vi "InputProc.vi"(7 "error in":errorcluster, 8 "output cluster":T15={[], {[], [], [], "GyroDevRef"={"DevStatus"={"status"=FALSE, "code"=0, "source"=""}, "Analog Channel"=enum."AI 0", "Offset"=0.0, "Gain (VoltsPerDegree/Second)"=0.0, "Gyro Type"=enum."Analog", "Handle"=0, "SPI Bus"=enum."Invalid", "Device Found"=FALSE, "Sample Rate"=1.0, "Calibrate On Open"=FALSE}, "CompressorDevRef"={"DevStatus"={"status"=FALSE, "code"=0, "source"=""}, "Pneumatics Control Module"=0}}} {"?"."GyroDevRef"."Sample Rate" min=0.25 max=100.0 step=0.25}, 9 "SensorInputData":T16, 10 "GamepadData":T17) -> (0 "error out":errorcluster, 2 "SensorInputDataOut":T16, 3 "GamepadDataOut":T17)   [LabVIEW 2015]
uses:
  Typedefs/GamepadData.ctl
  Typedefs/SensorInputData.ctl
  <vilib>/Rock Robotics/WPI/Joystick/WPI_JoystickDevRef.ctl
  <vilib>/Rock Robotics/WPI/Joystick/WPI_JoystickDeviceEnum.ctl
  <vilib>/Rock Robotics/WPI/Potentiometer/WPI_PotentiometerDevRef.ctl
  <vilib>/Rock Robotics/SystemInterfaces/AI/FPGA_AIChannel.ctl
  <vilib>/Rock Robotics/WPI/Encoder/WPI_EncoderDevRef.ctl
  <vilib>/Rock Robotics/SystemInterfaces/Encoder/FPGA_EncoderIdx.ctl
  <vilib>/Rock Robotics/SystemInterfaces/Counter/FPGA_CounterCtrSystemIndex.ctl
  <vilib>/Rock Robotics/WPI/Encoder/WPI_EncoderType.ctl
  <vilib>/Rock Robotics/WPI/Switch/WPI_SwitchDevRef.ctl
  <vilib>/Rock Robotics/SystemInterfaces/DIO/FPGA_DIOChannel.ctl
  <vilib>/Rock Robotics/WPI/Gyro/WPI_GyroDevRef.ctl
  <vilib>/Rock Robotics/SystemInterfaces/spilib/spi_bus.ctl
  <vilib>/Rock Robotics/WPI/Compressor/WPI_CompressorDevRef.ctl
  Gensubs/Bert_or_Ernie.vi
  Typedefs/JoysticksGlobal.vi
panel:
  in  "Wench Deadzone Limit":dbl=0.05 format="%#_13g"
  in  "X360 Deadzone Limit":dbl=0.3
  in  "Bert Arm Inputs":T1={"SensorMax"=0.929, "UnitMin"=-26.5, "SensorMin"=0.502, "UnitMax"=86.8}
  in  "Ernie Arm Inputs":T1={"SensorMax"=0.837, "UnitMin"=-26.7, "SensorMin"=0.444, "UnitMax"=87.4}
  out "Claw Pot Raw":dbl
  in  "Ernie StackerClamp Inputs":T1={"SensorMax"=0.852, "UnitMin"=148.3, "SensorMin"=0.477, "UnitMax"=219.6}
  in  "Ernie Stacker Inputs":T1={"SensorMax"=0.782, "UnitMin"=0.0, "SensorMin"=0.357, "UnitMax"=21.125}
  in  "Bert StackerClamp Inputs":T1={"SensorMax"=0.42, "UnitMin"=141.5, "SensorMin"=0.064, "UnitMax"=217.6}
  out "Stacker Clamp Pot Raw":dbl format="%#_13g"
  in  "F310 Deadzone Limit":dbl=0.05
  out "Arm Pot Raw":dbl
  out "Stacker Pot Raw":dbl
  in  "Bert Stacker Inputs":T1={"SensorMax"=0.501, "UnitMin"=0.0, "SensorMin"=0.082, "UnitMax"=21.125}
  in  "ENC_CPI":dbl=0.145
  # "is now f310"
  # "ENC_CPI is encoder counts per inch"
  # "Analog"
  # "XRS"
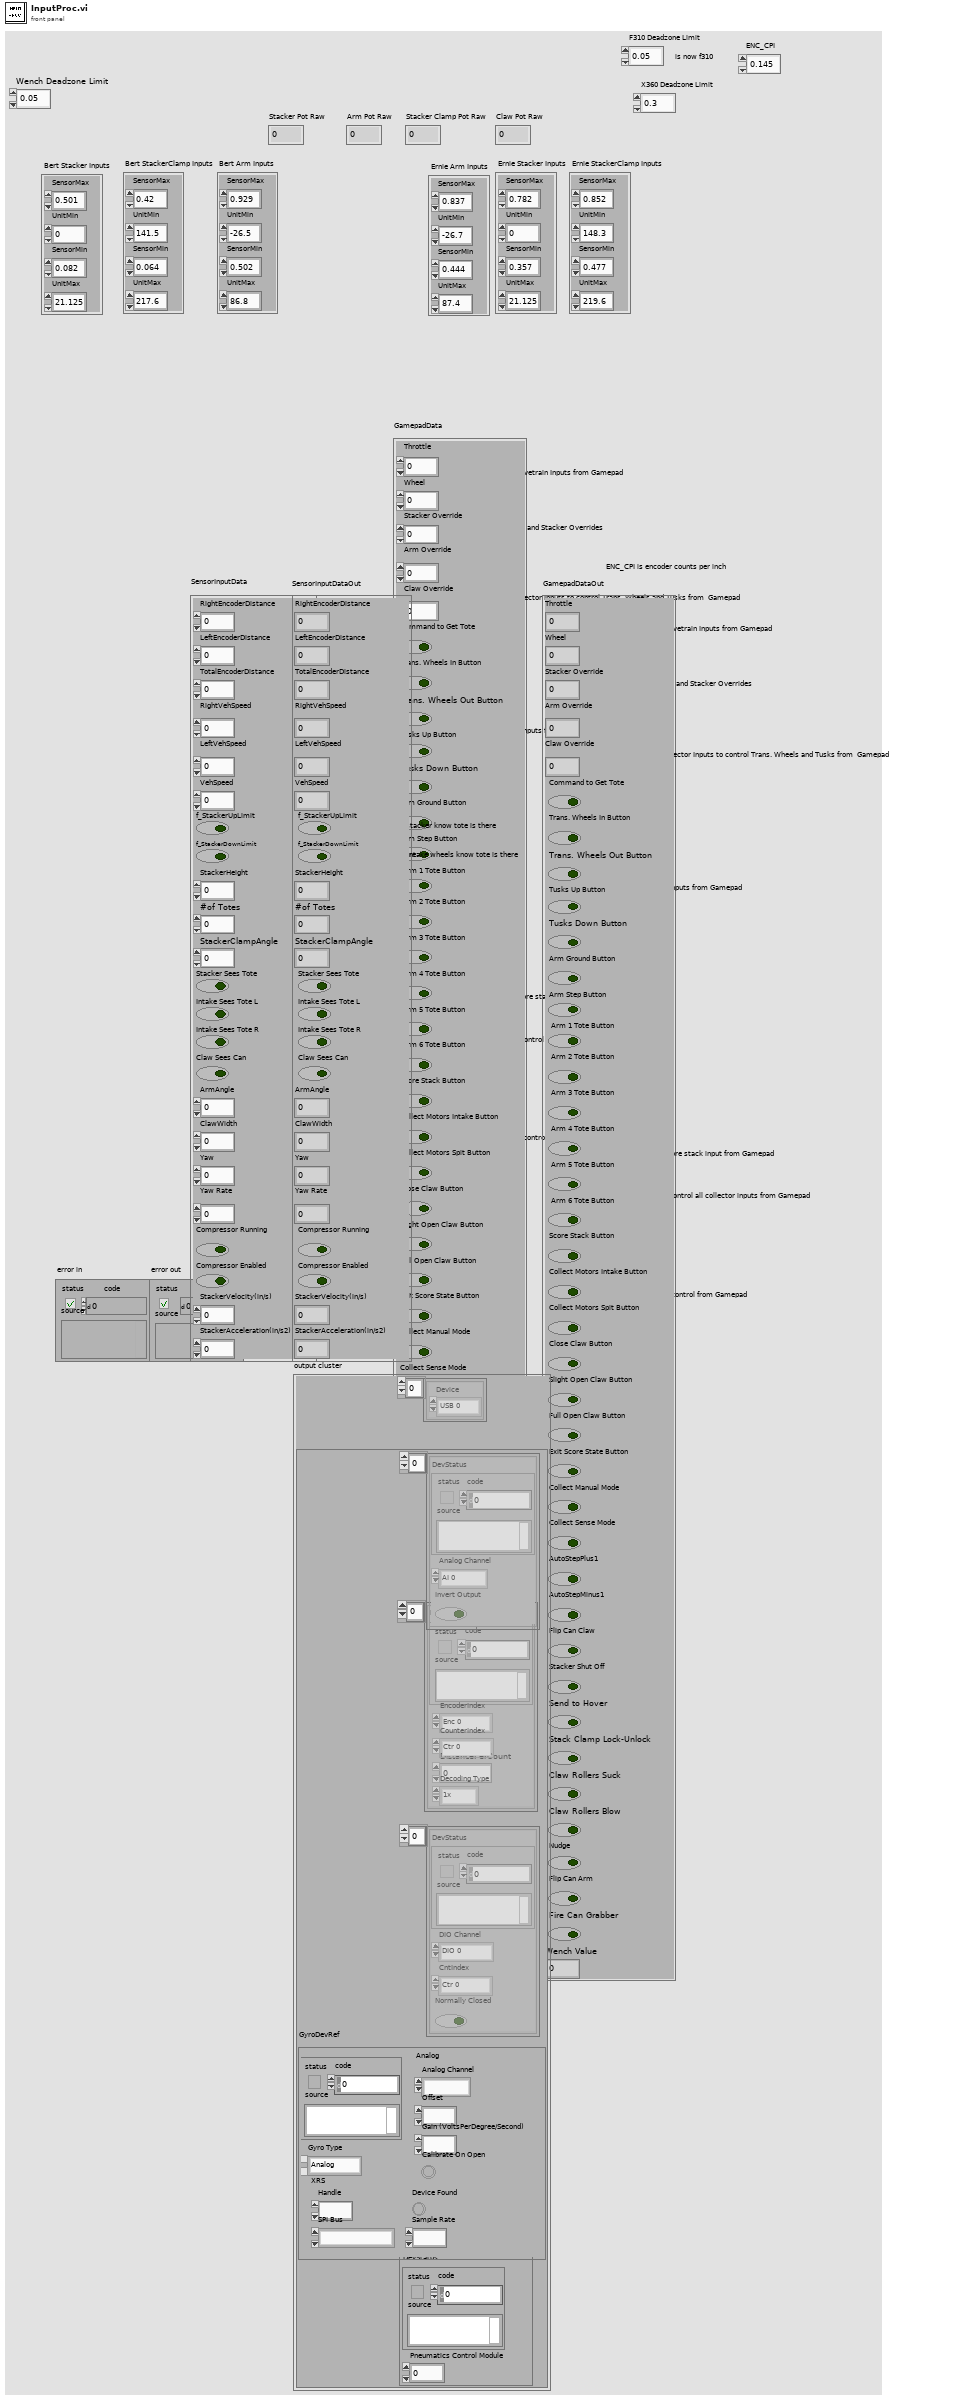
[diagram p1: front panel]
types:
  T1 = cluster{"SensorMax":dbl, "UnitMin":dbl, "SensorMin":dbl, "UnitMax":dbl}
  T2 = typedef "WPI_JoystickDevRef.ctl" = cluster{"Device":T3}
  T3 = typedef "WPI_JoystickDeviceEnum.ctl" = enum16{"USB 0", "USB 1", "USB 2", "USB 3", "USB 4", "USB 5"}
  T4 = typedef "WPI_PotentiometerDevRef.ctl" = cluster{"DevStatus":errorcluster, "Analog Channel":T5, "Invert Output":bool}
  T5 = typedef "FPGA_AIChannel.ctl" = enum8{"AI 0", "AI 1", "AI 2", "AI 3", "AI MXP 0", "AI MXP 1", "AI MXP 2", "AI MXP 3", "Invalid"}
  T6 = typedef "WPI_EncoderDevRef.ctl" = cluster{"DevStatus":errorcluster, "EncoderIndex":T7, "CounterIndex":T8, "DistancePerCount":dbl, "Decoding Type":T9}
  T7 = typedef "FPGA_EncoderIdx.ctl" = enum8{"Enc 0", "Enc 1", "Enc 2", "Enc 3", "Enc 4", "Enc 5", "Enc 6", "Enc 7", "Invalid"}
  T8 = typedef "FPGA_CounterCtrSystemIndex.ctl" = enum8{"Ctr 0", "Ctr 1", "Ctr 2", "Ctr 3", "Ctr 4", "Ctr 5", "Ctr 6", "Ctr 7", "Invalid"}
  T9 = typedef "WPI_EncoderType.ctl" = enum16{"1x", "2x", "4x"}
  T10 = typedef "WPI_SwitchDevRef.ctl" = cluster{"DevStatus":errorcluster, "DIO Channel":T11, "CntIndex":T8, "Normally Closed":bool}
  T11 = typedef "FPGA_DIOChannel.ctl" = enum8{"DIO 0", "DIO 1", "DIO 2", "DIO 3", "DIO 4", "DIO 5", "DIO 6", "DIO 7", "DIO 8", "DIO 9", "DIO MXP 0", "DIO MXP 1", "DIO MXP 2", "DIO MXP 3", "DIO MXP 4", "DIO MXP 5", "DIO MXP 6", "DIO MXP 7", "DIO MXP 8", "DIO MXP 9", "DIO MXP 10", "DIO MXP 11", "DIO MXP 12", "DIO MXP 13", "DIO MXP 14", "DIO MXP 15", "Invalid"}
  T12 = typedef "WPI_GyroDevRef.ctl" = cluster{"DevStatus":errorcluster, "Analog Channel":T5, "Offset":dbl, "Gain (VoltsPerDegree/Second)":dbl, "Gyro Type":enum16{"Analog", "XRS450"}, "Handle":i32, "SPI Bus":T13, "Device Found":bool, "Sample Rate":dbl, "Calibrate On Open":bool}
  T13 = typedef "spi_bus.ctl" = enum16{"SPI On-Board, CS0", "SPI On-Board, CS1", "SPI On-Board, CS2", "SPI On-Board, CS3", "SPI MXP", "Invalid"}
  T14 = typedef "WPI_CompressorDevRef.ctl" = cluster{"DevStatus":errorcluster, "Pneumatics Control Module":u8}
  T15 = cluster{T2[], cluster{T4[], T6[], T10[], "GyroDevRef":T12, "CompressorDevRef":T14}}
  T16 = typedef "SensorInputData.ctl" = cluster{"RightEncoderDistance":dbl, "LeftEncoderDistance":dbl, "TotalEncoderDistance":dbl, "RightVehSpeed":dbl, "LeftVehSpeed":dbl, "VehSpeed":dbl, "f_StackerUpLimit":bool, "f_StackerDownLimit":bool, "StackerHeight":dbl, "#of Totes":u8, "StackerClampAngle":dbl, "Stacker Sees Tote":bool, "Intake Sees Tote L":bool, "Intake Sees Tote R":bool, "Claw Sees Can":bool, "ArmAngle":dbl, "ClawWidth":dbl, "Yaw":dbl, "Yaw Rate":dbl, "Compressor Running":bool, "Compressor Enabled":bool, "StackerVelocity(in/s)":dbl, "StackerAcceleration(in/s2)":dbl}
  T17 = typedef "GamepadData.ctl" = cluster{"Throttle":dbl, "Wheel":dbl, "Stacker Override":dbl, "Arm Override ":dbl, "Claw Override":dbl, "Command to Get Tote":bool, "Trans. Wheels In Button":bool, "Trans. Wheels Out Button":bool, "Tusks Up Button":bool, "Tusks Down Button":bool, "Arm Ground Button":bool, "Arm Step Button":bool, " Arm 1 Tote Button":bool, " Arm 2 Tote Button":bool, " Arm 3 Tote Button ":bool, " Arm 4 Tote Button":bool, " Arm 5 Tote Button":bool, " Arm 6 Tote Button":bool, "Score Stack Button":bool, "Collect Motors Intake Button":bool, "Collect Motors Spit Button":bool, "Close Claw Button":bool, "Slight Open Claw Button":bool, "Full Open Claw Button ":bool, "Exit Score State Button":bool, "Collect Manual Mode ":bool, "Collect Sense Mode":bool, "AutoStepPlus1":bool, "AutoStepMinus1":bool, "Flip Can Claw":bool, "Stacker Shut Off":bool, "Send to Hover ":bool, "Stack Clamp Lock-Unlock ":bool, "Claw Rollers Suck ":bool, "Claw Rollers Blow ":bool, "Nudge":bool, "Flip Can Arm ":bool, "Fire Can Grabber":bool, "Wench Value":dbl}
  T18 = cluster{cluster{"Axes":dbl[], "Buttons":bool[], "POVs":i16[]}, cluster{"Axes":dbl[], "Buttons":bool[], "POVs":i16[]}, cluster{"Axes":dbl[], "Buttons":bool[], "POVs":i16[]}}
  T19 = cluster{T4[], T6[], T10[], "GyroDevRef":T12, "CompressorDevRef":T14}
  T20 = cluster{"Axes":dbl[], "Buttons":bool[], "POVs":i16[]}
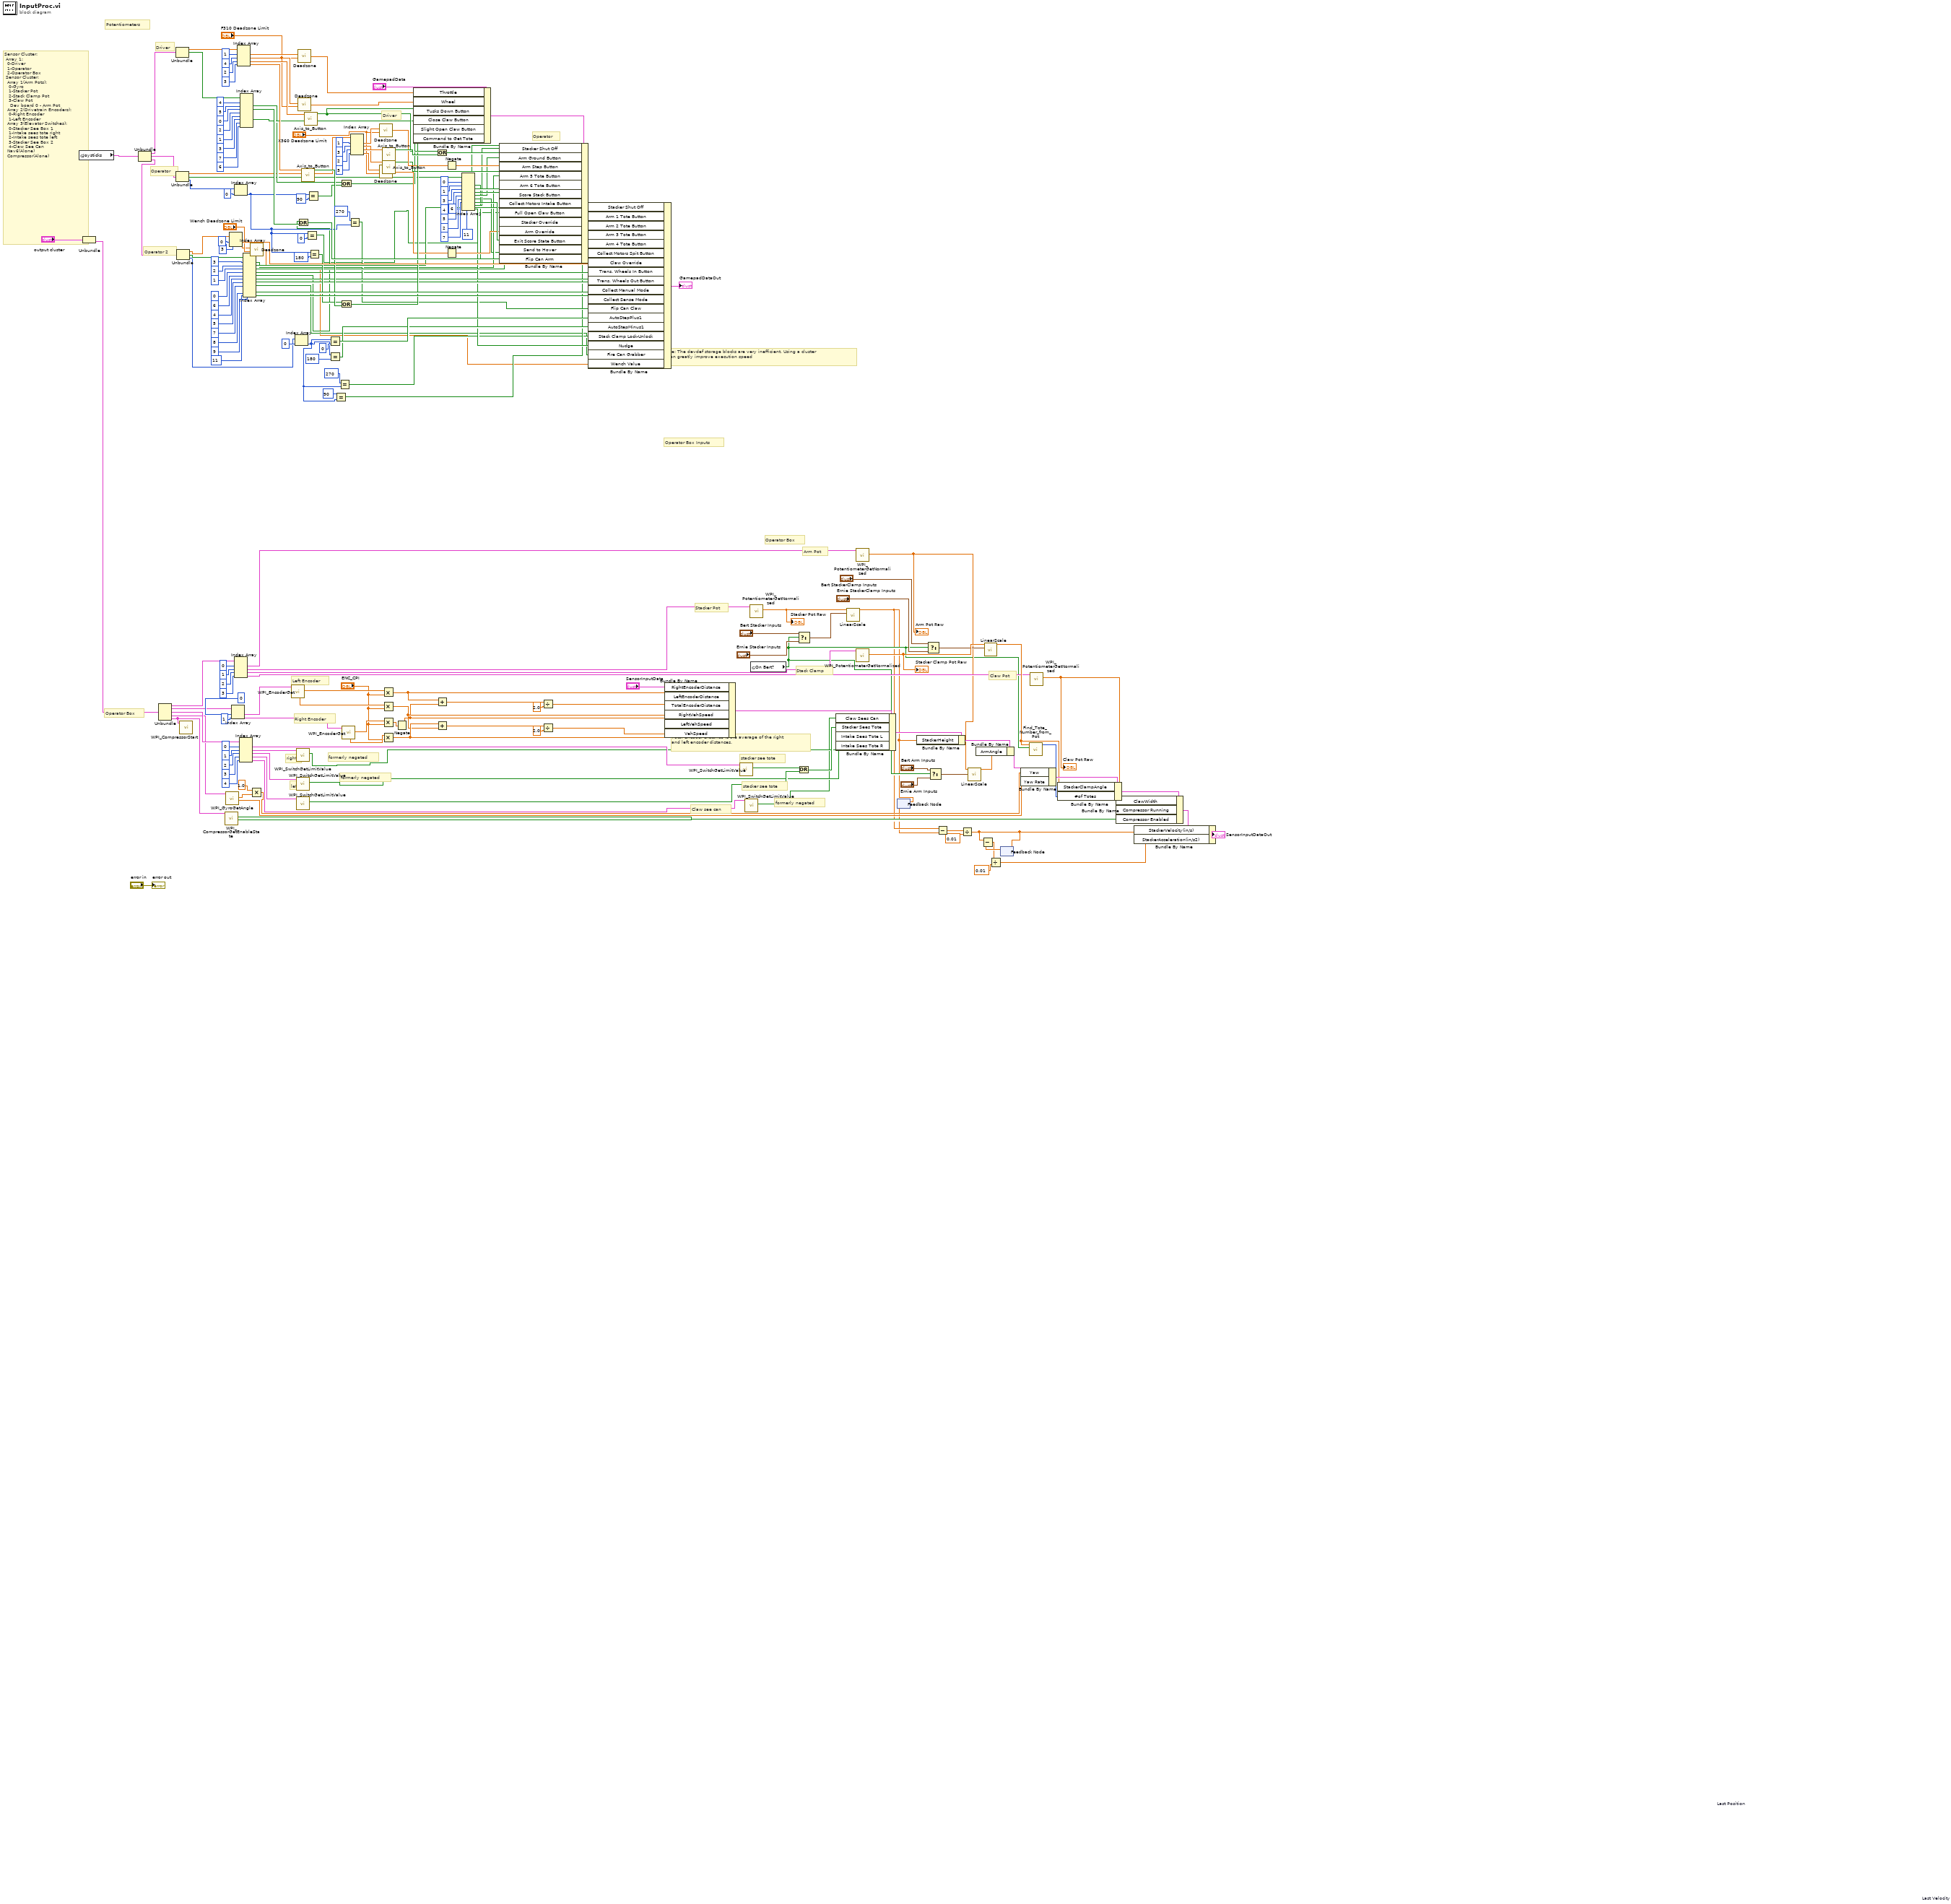
[diagram p0: block diagram]
diagram:
  # "formerly negated"
  # "right"
  # "formerly negated"
  # "formerly negated"
  # "Operator 2"
  # "Operator"
  # "Driver"
  # "Sensor Cluster:\n Array 1:\n  0-Driver\n  1-Operator\n  2-Operator Box\n Sensor Cluster:\n  Array 1(Arm Pots):\n   0-Gyro\n   1-Stacker Pot\n   2-Stack Clamp Pot\n   3-Claw Pot\n    Dev board 0 - Arm Pot\n  Array 2(Drivetrain Encoders):\n   0-Right Encoder\n   1-Left Encoder\n  Array 3(Elevator Switches):\n   0-Stacker See Box 1\n   1-Intake sees tote right\n   2-Intake sees tote left\n   3-Stacker See Box 2\n   4-Claw See Can \n  Nav6(Alone)\n  Compressor(Alone)"
  # "Claw see can"
  # "Claw Pot"
  # "stacker see tote"
  # "stacker see tote"
  # "Operator Box"
  # "Operator"
  # "Driver"
  # "Stack Clamp"
  # "Potentiometers"
  # "left"
  # "Operator Box"
  # "Operator Box Inputs"
  # "Arm Pot"
  # "Stacker Pot"
  # "Right Encoder"
  # "Left Encoder"
  # "Andrew's Note: The devdef storage blocks are very inefficient. Using a cluster\nof devdefs can greatly improve execution speed"
  # "Total Encoder Distance is the average of the right\nand left encoder distances."
  n1 = global read "JoysticksGlobal.vi" "Joysticks"() -> (w58:T18)
  n2 = Unbundle("output cluster") -> (w116:T19)  [unwired: 1 out]
  n3 = Unbundle(w58) -> (w57:T20, w51:T20, w46:T20)
  n4 = Unbundle(w116) -> (w196:T4[], w198:T6[], w191:T10[], "GyroDevRef"=w41:T12, "CompressorDevRef"=w115:T14)
  n5 = Unbundle(w57) -> ("Axes"=w56:dbl[], "Buttons"=w55:bool[])  [unwired: 1 out]
  n6 = Unbundle(w51) -> ("Axes"=w54:dbl[], "Buttons"=w53:bool[], "POVs"=w52:i16[])
  n7 = Unbundle(w46) -> ("Axes"=w50:dbl[], "Buttons"=w49:bool[], "POVs"=w48:i16[])
  n8 = call <vilib>:"WPI_CompressorStart.vi"("CompressorDevRef"=w115) -> ()  [unwired: 9 in, 2 out]
  n9 = call <vilib>:"WPI_CompressorGetEnableState.vi"("CompressorDevRef"=w115) -> ("Compressor Running"=w113:bool, "Enabled"=w114:bool)  [unwired: 7 in, 2 out]
  n10 = call <vilib>:"WPI_GyroGetAngle.vi"("GyroDevRef"=w41) -> ("Angular Rate"=w39:dbl, "Angle"=w40:dbl)  [unwired: 7 in, 2 out]
  n11 = Index Array(array=w50, index #1=0 ("index"), index #2=3 ("index")) -> (element #1=w120:dbl, element #2=w7:dbl)
  n12 = Index Array(array=w198, index #1=0 ("index"), index #2=1 ("index")) -> (element #1=w190:T6, element #2=w197:T6)
  n13 = Index Array(array=w52, index=0) -> (element=w23:i16)
  n14 = Index Array(array=w196, index #1=0 ("index"), index #2=1 ("index"), index #3=2 ("index"), index #4=3 ("index")) -> (element #1=w193:T4, element #2=w192:T4, element #3=w141:T4, element #4=w122:T4)
  n15 = Index Array(array=w56, index #1=1 ("index"), index #2=4 ("index"), index #3=2 ("index"), index #4=3 ("index")) -> (element #1=w159:dbl, element #2=w158:dbl, element #3=w180:dbl, element #4=w178:dbl)
  n16 = Index Array(array=w191, index #1=0 ("index"), index #2=1 ("index"), index #3=2 ("index"), index #4=3 ("index"), index #5=4 ("index")) -> (element #1=w163:T10, element #2=w155:T10, element #3=w154:T10, element #4=w151:T10, element #5=w118:T10)
  n17 = Index Array(array=w55, index #1=4 ("index"), index #2=5 ("index"), index #3=0 ("index"), index #4=2 ("index"), index #5=1 ("index"), index #6=3 ("index"), index #7=7 ("index"), index #8=6 ("index")) -> (element #2=w76:bool, element #3=w143:bool, element #6=w127:bool)  [unwired: 5 out]
  n18 = Index Array(array=w49, index #1=3 ("index"), index #2=2 ("index"), index #3=1 ("index"), index #4=0 ("index"), index #5=6 ("index"), index #6=4 ("index"), index #7=5 ("index"), index #8=7 ("index"), index #9=8 ("index"), index #10=9 ("index"), index #11=11 ("index")) -> (element #1=w15:bool, element #2=w42:bool, element #3=w38:bool, element #4=w16:bool, element #5=w11:bool, element #6=w75:bool, element #7=w74:bool, element #8=w10:bool, element #9=w94:bool, element #10=w92:bool)  [unwired: 1 out]
  n19 = call "Deadzone.vi"("Deadzone Limit"="Wench Deadzone Limit", "Value In"=w7) -> ("Value Out"=w6:dbl)  [unwired: 4 in]
  n20 = Multiply(x=1.0, y=w40) -> (x*y=w60:dbl)
  n21 = call <vilib>:"WPI_EncoderGet.vi"("EncoderDevRef"=w190) -> ("Distance"=w210:dbl, "Rate"=w107:dbl)  [unwired: 5 in, 4 out]
  n22 = Index Array(array=w48, index=0) -> (element=w22:i16)
  n23 = call <vilib>:"WPI_SwitchGetLimitValue.vi"("SwitchDevRef"=w155) -> ("Switch Pressed"=w5:bool)  [unwired: 8 in, 2 out]
  n24 = call <vilib>:"WPI_SwitchGetLimitValue.vi"("SwitchDevRef"=w154) -> ("Switch Pressed"=w4:bool)  [unwired: 8 in, 2 out]
  n25 = call <vilib>:"WPI_SwitchGetLimitValue.vi"("SwitchDevRef"=w151) -> ("Switch Pressed"=w148:bool)  [unwired: 8 in, 2 out]
  n26 = Or(x=w11, y=w143) -> (x .or. y?=w144:bool)
  n27 = call "Deadzone.vi"("Deadzone Limit"="F310 Deadzone Limit", "Value In"=w159) -> ("Value Out"=w160:dbl)  [unwired: 4 in]
  n28 = call "Deadzone.vi"("Deadzone Limit"="F310 Deadzone Limit", "Value In"=w158) -> ("Value Out"=w161:dbl)  [unwired: 4 in]
  n29 = call "Axis_to_Button.vi"("Axis"=w178) -> ("Signal"=w90:bool)  [unwired: 10 in]
  n30 = call "Axis_to_Button.vi"("Axis"=w180) -> ("Signal"=w145:bool)  [unwired: 10 in]
  n31 = Equal?(x=w23, y=i16 0) -> (x = y?=w3:bool)
  n32 = Equal?(x=w23, y=i16 90) -> (x = y?=w79:bool)
  n33 = Equal?(x=w23, y=i16 180) -> (x = y?=w77:bool)
  n34 = Equal?(x=w22, y=i16 0) -> (x = y?=w64:bool)
  n35 = Equal?(x=w22, y=i16 180) -> (x = y?=w63:bool)
  n36 = Equal?(x=i16 90 ("y"), y=w22) -> (x = y?=w13:bool)
  n37 = Equal?(x=i16 270 ("y"), y=w22) -> (x = y?=w12:bool)
  n38 = Or(x=w76, y=w79) -> (x .or. y?=w78:bool)
  n39 = Or(x=w77, y=w90) -> (x .or. y?=w89:bool)
  n40 = call <vilib>:"WPI_EncoderGet.vi"("EncoderDevRef"=w197) -> ("Distance"=w209:dbl, "Rate"=w108:dbl)  [unwired: 5 in, 4 out]
  n41 = Equal?(x=i16 270 ("y"), y=w23) -> (x = y?=w17:bool)
  n42 = Index Array(array=w54, index #1=1 ("index"), index #2=3 ("index"), index #3=2 ("index"), index #4=5 ("index")) -> (element #1=w85:dbl, element #2=w175:dbl, element #3=w176:dbl, element #4=w88:dbl)
  n43 = call "Deadzone.vi"("Deadzone Limit"="X360 Deadzone Limit", "Value In"=w85) -> ("Value Out"=w84:dbl)  [unwired: 4 in]
  n44 = call "Deadzone.vi"("Deadzone Limit"="X360 Deadzone Limit", "Value In"=w88) -> ("Value Out"=w87:dbl)  [unwired: 4 in]
  n45 = Multiply(x=w210, y="ENC_CPI") -> (x*y=w45:dbl)
  n46 = Multiply(x=w107, y="ENC_CPI") -> (x*y=w105:dbl)
  n47 = Multiply(x=w209, y="ENC_CPI") -> (x*y=w44:dbl)
  n48 = Multiply(x=w108, y="ENC_CPI") -> (x*y=w106:dbl)
  n49 = call "Axis_to_Button.vi"("Axis"=w176) -> ("Signal"=w146:bool)  [unwired: 10 in]
  n50 = call "Axis_to_Button.vi"("Axis"=w175) -> ("Signal"=w82:bool)  [unwired: 10 in]
  n51 = Negate(x=w44) -> (-x=w43:dbl)
  n52 = Bundle By Name(cluster="GamepadData", "Throttle"=w160, "Wheel"=w161, "Tusks Down Button"=w145, "Close Claw Button"=w89, "Slight Open Claw Button"=w78, "Command to Get Tote"=w127) -> (w213:T17)
  n53 = Or(x=w145, y=w146) -> (x .or. y?=w147:bool)
  n54 = Add(x=w45, y=w43) -> (x+y=w207:dbl)
  n55 = Add(x=w106, y=w105) -> (x+y=w104:dbl)
  n56 = Negate(x=w84) -> (-x=w100:dbl)
  n57 = Negate(x=w87) -> (-x=w99:dbl)
  n58 = Index Array(array=w53, index #1=0 ("index"), index #2=1 ("index"), index #3=3 ("index"), index #4=4 ("index"), index #5=5 ("index"), index #6=2 ("index"), index #7=7 ("index"), index #8=11 ("index"), index #9=6 ("index")) -> (element #1=w20:bool, element #2=w19:bool, element #3=w170:bool, element #4=w83:bool, element #5=w81:bool, element #6=w14:bool, element #7=w166:bool, element #8=w61:bool, element #9=w18:bool)
  n59 = Bundle By Name(cluster=w213, "Stacker Shut Off"=w61, "Arm Ground Button"=w81, "Arm Step Button"=w82, "Arm 5 Tote Button"=w15, "Arm 6 Tote Button"=w170, "Score Stack Button"=w83, "Collect Motors Intake Button"=w147, "Full Open Claw Button"=w3, "Stacker Override"=w100, "Arm Override"=w99, "Exit Score State Button"=w166, "Send to Hover"=w38, "Flip Can Arm"=w19) -> (w184:T17)
  n60 = Divide(x=w207, y=2.0) -> (x/y=w206:dbl)
  n61 = Divide(x=w104, y=2.0) -> (x/y=w103:dbl)
  n62 = Bundle By Name(cluster=w184, "Stacker Shut Off"=w42, "Arm 1 Tote Button"=w20, "Arm 2 Tote Button"=w13, "Arm 3 Tote Button"=w14, "Arm 4 Tote Button"=w16, "Collect Motors Spit Button"=w144, "Claw Override"=w120, "Trans. Wheels In Button"=w75, "Trans. Wheels Out Button"=w74, "Collect Manual Mode"=w94, "Collect Sense Mode"=w92, "Flip Can Claw"=w17, "AutoStepPlus1"=w64, "AutoStepMinus1"=w63, "Stack Clamp Lock-Unlock"=w12, "Nudge"=w18, "Fire Can Grabber"=w10, "Wench Value"=w6) -> (→"GamepadDataOut":T17)
  n63 = Bundle By Name(cluster="SensorInputData", "RightEncoderDistance"=w43, "LeftEncoderDistance"=w45, "TotalEncoderDistance"=w206, "RightVehSpeed"=w105, "LeftVehSpeed"=w106, "VehSpeed"=w103) -> (w204:T16)
  n64 = call <vilib>:"WPI_SwitchGetLimitValue.vi"("SwitchDevRef"=w163) -> ("Switch Pressed"=w150:bool)  [unwired: 8 in, 2 out]
  n65 = call <vilib>:"WPI_SwitchGetLimitValue.vi"("SwitchDevRef"=w118) -> ("Switch Pressed"=w2:bool)  [unwired: 8 in, 2 out]
  n66 = call <vilib>:"WPI_PotentiometerGetNormalized.vi"("PotDevRef"=w192) -> ("Normalized Value"=w182:dbl)  [unwired: 8 in, 2 out]
  "Stacker Pot Raw" <- w182
  n67 = global read "Bert_or_Ernie.vi" "On Bert?"() -> (w68:bool)
  n68 = Select(t="Bert Stacker Inputs", s=w68, f="Ernie Stacker Inputs") -> (s? t:f=w131:T1)
  n69 = Or(x=w150, y=w148) -> (x .or. y?=w149:bool)
  n70 = Bundle By Name(cluster=w204, "Claw Sees Can"=w2, "Stacker Sees Tote"=w149, "Intake Sees Tote L"=w4, "Intake Sees Tote R"=w5) -> (w203:T16)
  n71 = call "LinearScale.vi"("RawInput"=w182, "UnitsPlease Inputs"=w131) -> ("UnitOutput"=w34:dbl)  [unwired: 13 in]
  n72 = call <vilib>:"WPI_PotentiometerGetNormalized.vi"("PotDevRef"=w193) -> ("Normalized Value"=w73:dbl)  [unwired: 8 in, 2 out]
  "Arm Pot Raw" <- w73
  n73 = call <vilib>:"WPI_PotentiometerGetNormalized.vi"("PotDevRef"=w141) -> ("Normalized Value"=w140:dbl)  [unwired: 8 in, 2 out]
  "Stacker Clamp Pot Raw" <- w140
  n74 = feedback-in #1(w34) -> ()
  n75 = feedback #1 "Last Position"() -> (w33:dbl)  [unwired: 1 in]
  n76 = Bundle By Name(cluster=w203, "StackerHeight"=w34) -> (w202:T16)
  n77 = Select(t="Bert StackerClamp Inputs", s=w68, f="Ernie StackerClamp Inputs") -> (s? t:f=w135:T1)
  n78 = Select(t="Bert Arm Inputs", s=w68, f="Ernie Arm Inputs") -> (s? t:f=w70:T1)
  n79 = Subtract(x=w34, y=w33) -> (x-y=w31:dbl)
  n80 = Divide(x=w31, y=0.01) -> (x/y=w30:dbl)
  n81 = call "LinearScale.vi"("RawInput"=w73, "UnitsPlease Inputs"=w70) -> ("UnitOutput"=w72:dbl)  [unwired: 13 in]
  n82 = Bundle By Name(cluster=w202, "ArmAngle"=w72) -> (w201:T16)
  n83 = call "LinearScale.vi"("RawInput"=w140, "UnitsPlease Inputs"=w135) -> ("UnitOutput"=w137:dbl)  [unwired: 13 in]
  n84 = feedback #2 "Last Velocity"() -> (w29:dbl)  [unwired: 1 in]
  n85 = Subtract(x=w30, y=w29) -> (x-y=w28:dbl)
  n86 = Divide(x=w28, y=0.01) -> (x/y=w26:dbl)
  n87 = feedback-in #2(w30) -> ()
  n88 = Bundle By Name(cluster=w201, "Yaw"=w60, "Yaw Rate"=w39) -> (w139:T16)
  n89 = call "Find_Tote_Number_from_Pot.vi"("On Bert?"=w68, "Stack Clamp Angle"=w137) -> ("Number of Totes"=w138:i8)  [unwired: 9 in]
  n90 = call <vilib>:"WPI_PotentiometerGetNormalized.vi"("PotDevRef"=w122) -> ("Normalized Value"=w117:dbl)  [unwired: 8 in, 2 out]
  "Claw Pot Raw" <- w117
  n91 = Bundle By Name(cluster=w139, "StackerClampAngle"=w137, "#of Totes"=w138) -> (w123:T16)
  n92 = Bundle By Name(cluster=w123, "ClawWidth"=w117, "Compressor Running"=w113, "Compressor Enabled"=w114) -> (w36:T16)
  n93 = Bundle By Name(cluster=w36, "StackerVelocity(in/s)"=w30, "StackerAcceleration(in/s2)"=w26) -> (→"SensorInputDataOut":T16)
  "error out" <- "error in"
